vi "BotSpeak_Stepper.vi"(2 "DIO Line":u8(slide) scale=0.0..3.0, 3 "# pulses":u32=2, 4 "Bot Settings":T1) -> (0 "response":string="169.254.32.85", 1 "Bot Settings 2":T1)   [LabVIEW 2014]
doc: "Drives a stepper motor via the RIO. Given the \"DIO line\" to which the stepper is wired, the stepper will turn the specified \"number of pulses\"."
uses:
  <userlib>/botspeak/VIs/Direct/BotSpeak_Control.ctl
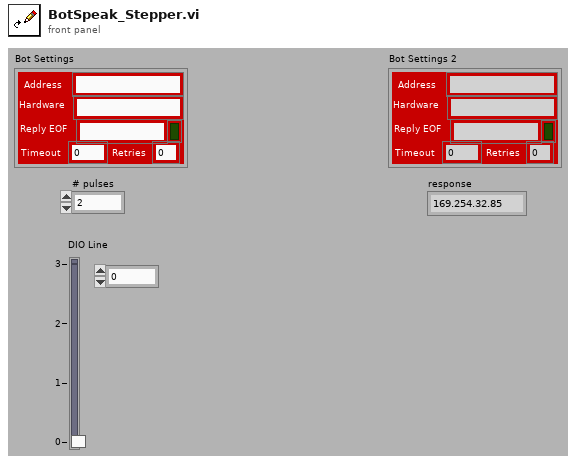
[diagram p1: front panel]
types:
  T1 = typedef "BotSpeak_Control.ctl" = cluster{"Address":string, "Reply EOF":string, "Hardware":string, "Retries":i8, "Timeout":i32, "Open?":bool}
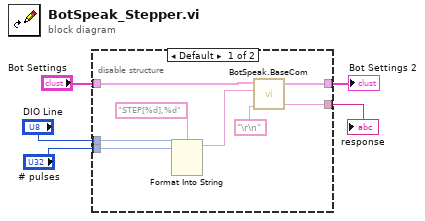
[diagram p0: block diagram]
diagram:
  n1 = disable-structure shown="Default" {
    disable-tunnel: "DIO Line" -> [w13 _]
    disable-tunnel: "# pulses" -> [w12 _]
    disable-tunnel: "Bot Settings" -> [w9 _]
    disable-tunnel: [w8 _] -> w2
    disable-tunnel: [w6 _] -> w1
    frame condition #0 {
      n2 = Format Into String(format string="STEP[%d],%d" ("command"), w13, w12) -> (resulting string=w7:string)  [unwired: 2 in, 1 out]
      n3 = call <userlib>:"BotSpeak.BaseCom.vi"("Termination"="\r\n", "command"=w7, "Bot Settings in"=w9) -> ("response"=w6:string, "Bot Settings out"=w8:T1)  [unwired: 2 in]
    }
    frame condition #1 (active) {
    }
  }
  "Bot Settings 2" <- w2
  "response" <- w1
